vi "Process Notifiers and Queue.vi"(8 "error in (no error)":errorcluster, 10 "cluster":T2, 11 "DAQmx":refnum<class "DAQmx.lvclass">) -> (0 "error out":errorcluster, 1 "AOwfm":waveform(dbl)[](array[waveform]), 2 "State":T1, 3 "DAQmx out":refnum<class "DAQmx.lvclass">)   [LabVIEW 2019, in "DAQmx.lvclass"]
uses:
  DAQmx.lvclass
  typedefs/DAQmx.States--enum.ctl
  typedefs/DAQ.Config.AO--Cluster--Array.ctl
  typedefs/DAQ.Config.AO--Cluster.ctl
  typedefs/DAQ.Config.AO.Range--enum.ctl
  typedefs/DAQ.Config.Device Type--enum.ctl
  typedefs/DAQ.Config.AI--Cluster--Array.ctl
  typedefs/DAQ.Config.AI--Cluster.ctl
  typedefs/DAQ.Config.AI.Coupling--enum.ctl
  typedefs/DAQ.Config.AI.Range--enum.ctl
  typedefs/DAQ.Config.Timing--Cluster.ctl
  typedefs/DAQ.Config.Timing.Sampling--Cluster.ctl
  typedefs/DAQ.Config.Timing.Fs Mode--enum.ctl
  DAQmx.lvclass/DAQmx.ctl
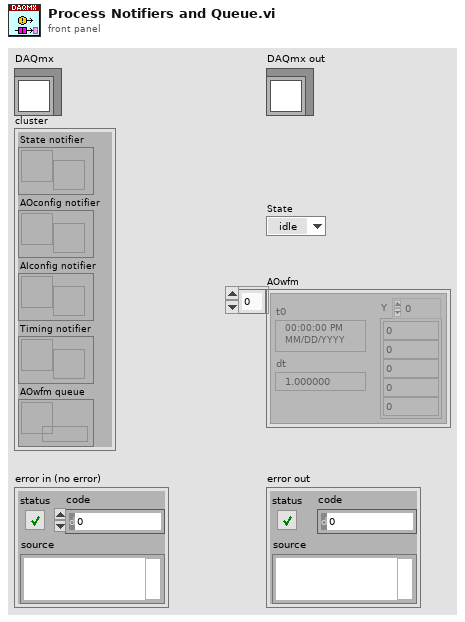
[diagram p1: front panel]
types:
  T1 = typedef "DAQmx.lvclass/DAQmx.States--enum.ctl" = enum16{"idle", "start", "stop", "calibrate", "auto"}
  T2 = cluster{"State notifier":refnum<notifier>, "AOconfig notifier":refnum<notifier>, "AIconfig notifier":refnum<notifier>, "Timing notifier":refnum<notifier>, "AOwfm queue":refnum<queue>}
  T3 = typedef "DAQmx.lvclass/DAQ.Config.Timing--Cluster.ctl" = cluster{"Sampling":T4, "sample mode":i32, "FsMode":T5, "Fs Multiplier":dbl, "Refresh Rate (Hz)":dbl, "Decimation.PreDSP":i32, "Decimation.PostDSP":i32, "Fs.Output":dbl}
  T4 = typedef "DAQmx.lvclass/DAQ.Config.Timing.Sampling--Cluster.ctl" = cluster{"Fs":dbl, "#s":i32}
  T5 = typedef "DAQmx.lvclass/DAQ.Config.Timing.Fs Mode--enum.ctl" = enum16{"Manual", "Auto Fs", "Max Fs"}
  T6 = typedef "DAQmx.lvclass/DAQ.Config.AI--Cluster--Array.ctl" = T7[]
  T7 = typedef "DAQmx.lvclass/DAQ.Config.AI--Cluster.ctl" = cluster{"Channels":tag, "Coupling":T8, "Range":T9, "input terminal configuration":i32, "Type":T10}
  T8 = typedef "DAQmx.lvclass/DAQ.Config.AI.Coupling--enum.ctl" = u16
  T9 = typedef "DAQmx.lvclass/DAQ.Config.AI.Range--enum.ctl" = enum16{"±0.316", "±1.00", "±3.16", "±10.0", "±31.6", "±42.4", ""}
  T10 = typedef "DAQmx.lvclass/DAQ.Config.Device Type--enum.ctl" = enum16{"None", "USB-4431", "PXI-446x"}
  T11 = typedef "DAQmx.lvclass/DAQ.Config.AO--Cluster--Array.ctl" = T12[]
  T12 = typedef "DAQmx.lvclass/DAQ.Config.AO--Cluster.ctl" = cluster{"Channels":tag, "Range":T13, "output terminal configuration":i32, "Type":T10}
  T13 = typedef "DAQmx.lvclass/DAQ.Config.AO.Range--enum.ctl" = enum16{"±0.1", "±1.0", "±10.0", ""}
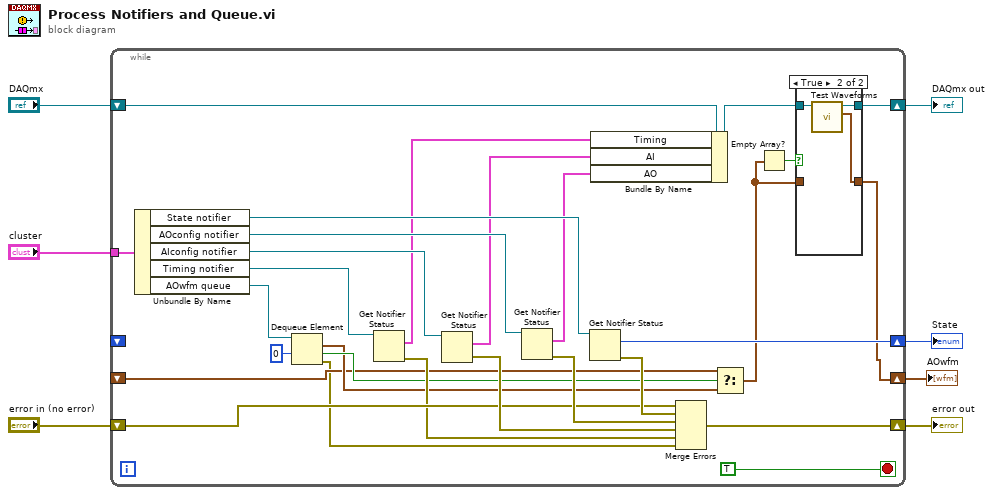
[diagram p0: block diagram]
diagram:
  n1 = while {
    tunnel: "cluster" -> [w35]
    shift-right: [w11] -> w5
    shift-left: "DAQmx" -> [w29]
    shift-right: [w20] -> w3
    shift-left: "error in (no error)" -> [w22]
    shift-right: [w8] -> w1
    shift-left: _ -> [w15]
    shift-right: [w13] -> w2
    shift-left: _ -> [_]
    stop <- TRUE stop-if-true
    n2 = Unbundle By Name(w35) -> ("State notifier"=w31:refnum<notifier>, "AOconfig notifier"=w32:refnum<notifier>, "AIconfig notifier"=w33:refnum<notifier>, "Timing notifier"=w34:refnum<notifier>, "AOwfm queue"=w30:refnum<queue>)
    n3 = Dequeue Element(queue=w30, timeout in ms (-1)=0) -> (element=w16:waveform(dbl)[], timed out?=w17:bool, error out=w14:errorcluster)  [unwired: 1 in, 1 out]
    n4 = Get Notifier Status(notifier=w34) -> (current notification=w26:T3, error out=w21:errorcluster)  [unwired: 1 in, 3 out]
    n5 = Get Notifier Status(notifier=w33) -> (current notification=w27:T6, error out=w23:errorcluster)  [unwired: 1 in, 3 out]
    n6 = Get Notifier Status(notifier=w32) -> (current notification=w28:T11, error out=w24:errorcluster)  [unwired: 1 in, 3 out]
    n7 = Get Notifier Status(notifier=w31) -> (current notification=w13:T1, error out=w25:errorcluster)  [unwired: 1 in, 3 out]
    n8 = Bundle By Name(cluster=w29, "Timing"=w26, "AI"=w27, "AO"=w28) -> (w12:refnum<class "DAQmx.lvclass">)
    n9 = Merge Errors(w22, w25, w24, w23, w21, w14) -> (w20:errorcluster)
    n10 = Select(t=w15, s=w17, f=w16) -> (s? t:f=w9:waveform(dbl)[])
    n11 = Empty Array?(array=w9) -> (empty?=w10:bool)
    n12 = case shown="True" w10 {
      tunnel: w12 -> [w36 w40]
      tunnel: [w36 w39] -> w11
      tunnel: [w37 w38] -> w8
      tunnel: w9 -> [w37 _]
      frame False {
      }
      frame True {
        n13 = call "Test Waveforms.vi"("DAQmx in"=w40) -> ("Array"=w38:waveform(dbl)[], "DAQmx out"=w39:refnum<class "DAQmx.lvclass">)  [unwired: 8 in, 1 out]
      }
    }
  }
  "error out" <- w3
  "DAQmx out" <- w5
  "State" <- w2
  "AOwfm" <- w1
